vi "Cook dinner.vi"() -> ()   [LabVIEW 2020]
uses:
  Chef/Chef.lvclass
  Microwave/Microwave.lvclass
  D:/LabVIEW/LabVIEW codes/solutions_and_repetitions/Strategy_pattern/Appliance/Appliance.lvclass
  Toaster/Toaster.lvclass
  Oven/Oven.lvclass
panel:
  in  "Select Appliance":string(combo)
  in  "stop":bool
  in  "Toast":bool
  in  "Steam":bool
  in  "Broil":bool
  in  "Braise":bool
  in  "Bake":bool
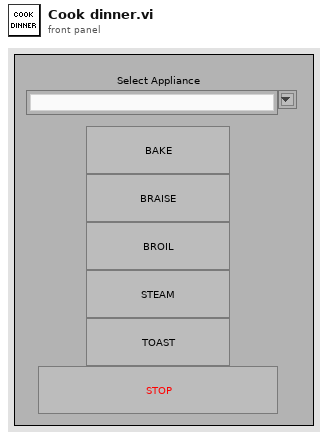
[diagram p1: front panel]
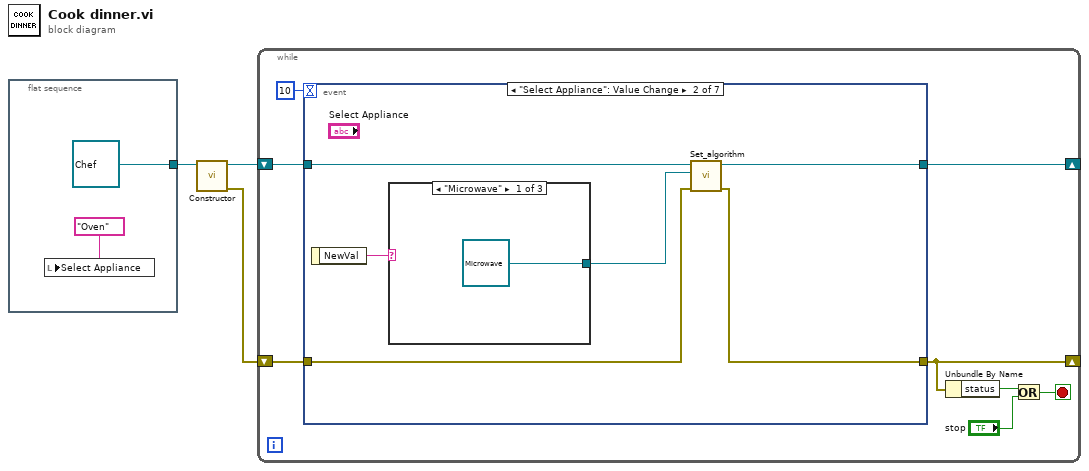
[diagram p0: block diagram]
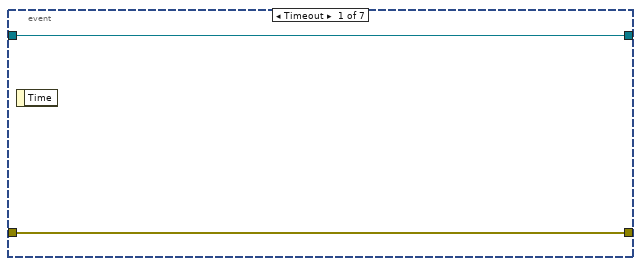
[diagram p2: hidden frame]
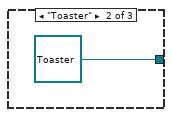
[diagram p3: hidden frame]
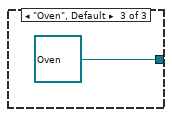
[diagram p4: hidden frame]
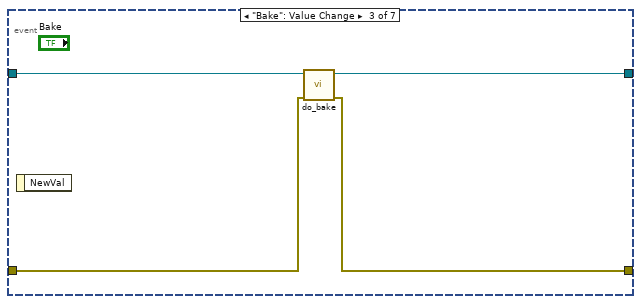
[diagram p5: hidden frame]
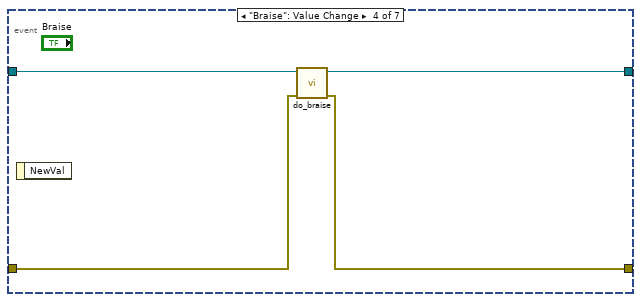
[diagram p6: hidden frame]
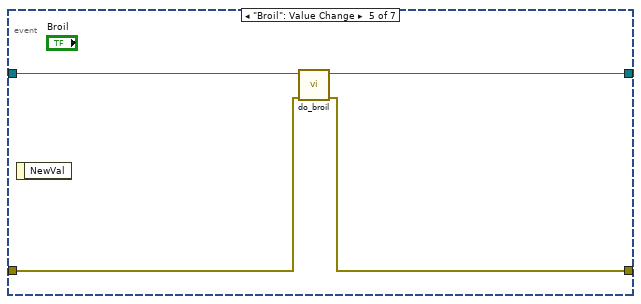
[diagram p7: hidden frame]
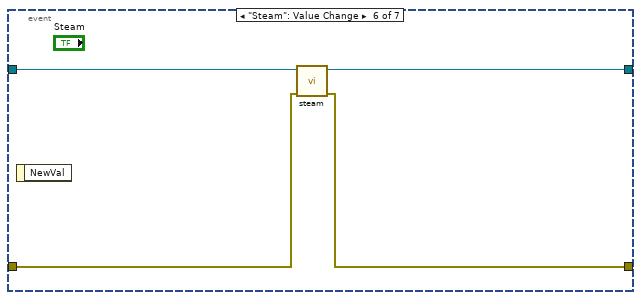
[diagram p8: hidden frame]
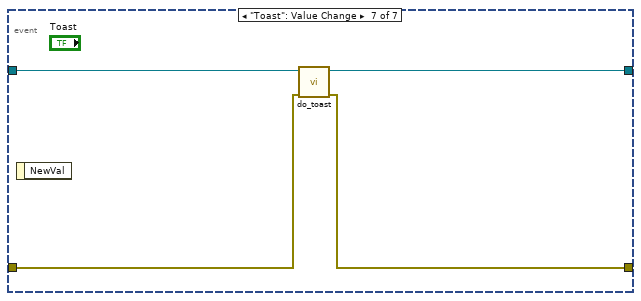
[diagram p9: hidden frame]
diagram:
  n1 = flat-sequence {
    tunnel: [refnum<class "Chef.lvclass"> refnum ("Chef.lvclass")] -> w3
    frame #0 {
      n2 = local write "Select Appliance"("Oven" ("Select Appliance")) -> ()
    }
  }
  n3 = call-dynamic "Constructor.vi"("Chef in"=w3) -> ("error out"=w1:errorcluster, "Chef out"=w2:refnum<class "Chef.lvclass">)  [unwired: 9 in]
  n4 = while {
    shift-right: [w11] -> _
    shift-left: w2 -> [w12]
    shift-right: [w9] -> _
    shift-left: w1 -> [w10]
    stop <- w6 stop-if-true
    n5 = event shown="[1] \"Select Appliance\": Value Change" {
      selector: _ -> [_ _ _ _ _ _ _]
      dyn-events: _ -> [_ _ _ _ _ _ _]
      timeout: 10 -> [_ _ _ _ _ _ _]
      tunnel: w12 -> [w15 w21 w28 w32 w36 w40 w44]
      tunnel: [w15 w20 w27 w31 w35 w39 w43] -> w11
      tunnel: w10 -> [w14 w19 w26 w30 w34 w38 w42]
      tunnel: [w14 w18 w25 w29 w33 w37 w41] -> w9
      event Timeout {
        n6 = event-data() -> ()  [unwired: 1 in, 1 out]
      }
      event "Select Appliance": Value Change {
        n7 = event-data() -> ("NewVal"=w17:string)  [unwired: 1 in]
        n8 = case shown="\"Microwave\"" w17 {
          tunnel: [refnum<class "Microwave.lvclass"> refnum ("Microwave.lvclass") refnum<class "Toaster.lvclass"> refnum ("Toaster.lvclass") refnum<class "Oven.lvclass"> refnum ("Oven.lvclass")] -> w16
          frame "Microwave" {
          }
          frame "Toaster" {
          }
          frame "Oven", Default {
          }
        }
        n9 = call-dynamic "Set_algorithm.vi"("error in (no error)"=w19, "Appliance.lvclass"=w16, "Chef in"=w21) -> ("error out"=w18:errorcluster, "Chef out"=w20:refnum<class "Chef.lvclass">)  [unwired: 7 in]
      }
      event "Bake": Value Change {
        n10 = event-data() -> ()  [unwired: 1 in, 1 out]
        n11 = call-dynamic "do_bake.vi"("error in (no error)"=w26, "Chef in"=w28) -> ("error out"=w25:errorcluster, "Chef out"=w27:refnum<class "Chef.lvclass">)  [unwired: 8 in]
      }
      event "Braise": Value Change {
        n12 = event-data() -> ()  [unwired: 1 in, 1 out]
        n13 = call-dynamic "do_braise.vi"("error in (no error)"=w30, "Chef in"=w32) -> ("error out"=w29:errorcluster, "Chef out"=w31:refnum<class "Chef.lvclass">)  [unwired: 8 in]
      }
      event "Broil": Value Change {
        n14 = event-data() -> ()  [unwired: 1 in, 1 out]
        n15 = call-dynamic "do_broil.vi"("error in (no error)"=w34, "Chef in"=w36) -> ("error out"=w33:errorcluster, "Chef out"=w35:refnum<class "Chef.lvclass">)  [unwired: 8 in]
      }
      event "Steam": Value Change {
        n16 = event-data() -> ()  [unwired: 1 in, 1 out]
        n17 = call-dynamic "steam.vi"("error in (no error)"=w38, "Chef in"=w40) -> ("error out"=w37:errorcluster, "Chef out"=w39:refnum<class "Chef.lvclass">)  [unwired: 8 in]
      }
      event "Toast": Value Change {
        n18 = event-data() -> ()  [unwired: 1 in, 1 out]
        n19 = call-dynamic "do_toast.vi"("error in (no error)"=w42, "Chef in"=w44) -> ("error out"=w41:errorcluster, "Chef out"=w43:refnum<class "Chef.lvclass">)  [unwired: 8 in]
      }
    }
    n20 = Unbundle By Name(w9) -> ("status"=w8:bool)
    n21 = Or(x=w8, y="stop") -> (x .or. y?=w6:bool)
  }
